vi "Pull Behavior_MWMATHIS.vi"(7 "Water Reward File":path=path "C:/Users/Mackenzie Amoroso/Desktop/REWARD_ente7102015") -> ()   [LabVIEW 2012] (continued)
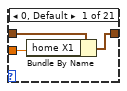
[diagram p2: hidden frame]
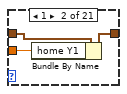
[diagram p3: hidden frame]
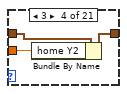
[diagram p4: hidden frame]
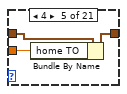
[diagram p5: hidden frame]
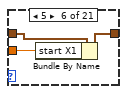
[diagram p6: hidden frame]
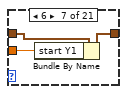
[diagram p7: hidden frame]
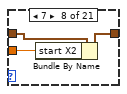
[diagram p8: hidden frame]
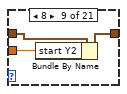
[diagram p9: hidden frame]
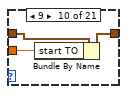
[diagram p10: hidden frame]
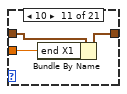
[diagram p11: hidden frame]
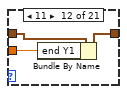
[diagram p12: hidden frame]
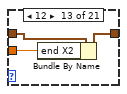
[diagram p13: hidden frame]
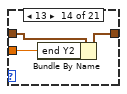
[diagram p14: hidden frame]
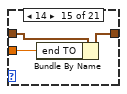
[diagram p15: hidden frame]
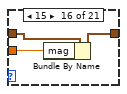
[diagram p16: hidden frame]
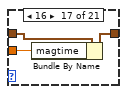
[diagram p17: hidden frame]
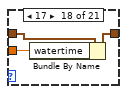
[diagram p18: hidden frame]
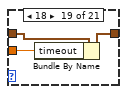
[diagram p19: hidden frame]
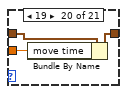
[diagram p20: hidden frame]
        n161 = Write to Binary File(file (use dialog)=w292, data=w283, 5:w279) -> (refnum out=w281:refnum<file>)  [unwired: 3 in, 2 out]
        n162 = local read "frame count 2"() -> (w278:u32)
        n163 = To Single Precision Float(number=w278) -> (single precision float=w277:sgl)
        n164 = Write to Binary File(file (use dialog)=w281, data=w277, 5:FALSE ("prepend array or string size? (T)")) -> (refnum out=w280:refnum<file>)  [unwired: 3 in, 2 out]
        n165 = local read "trial queue"() -> (w288:refnum<queue>)
        n166 = Dequeue Element(queue=w288) -> (element=w287:i32)  [unwired: 2 in, 3 out]
        n167 = To Single Precision Float(number=w287) -> (single precision float=w289:sgl)
        n168 = Write to Binary File(file (use dialog)=w280, data=w289, 5:w279) -> (refnum out=w290:refnum<file>)  [unwired: 3 in, 2 out]
        n169 = node-c288(w294) -> ()  [unwired: 1 out]
      }
      frame True {
      }
    }
    n170 = local read "stop"() -> (w275:bool)
  }
  n171 = local read "exp para array"() -> (w8:T1)
  n172 = while {
    tunnel: w30 -> [w328]
    tunnel: w27 -> [w331]
    tunnel: [w330] -> w26
    tunnel: w8 -> [w325]
    stop <- w332 stop-if-true
    # "on occurance signal give water"
    n173 = Wait on Occurrence(1:TRUE ("ignore previous (T)"), 2:w328, 3:100 ("ms timeout (-1)")) -> (0:w329:bool)
    n174 = local read "Trial #"() -> (w324:dbl)
    n175 = Index Array(array=w325, index=w324) -> (element=w323:T2)
    n176 = Unbundle By Name(w323) -> ("watertime"=w322:dbl)
    n177 = case shown="False" w329 {
      tunnel: w331 -> [w335 w361]
      tunnel: [w334 w361] -> w330
      tunnel: w322 -> [w333 _]
      frame False {
        n178 = node-c288() -> (w337:T4)  [unwired: 4 in]
        n179 = timed-sequence {
          timing: w337 -> [_]
          timing-out: [_] -> w336
          tunnel: w335 -> [w340]
          tunnel: [w339] -> w334
          tunnel: w333 -> [w338]
          n180 = timed-flat-sequence {
            tunnel: w340 -> [w348]
            tunnel: [w343] -> w339
            tunnel: w338 -> [w345]
            frame #0 {
              n181 = node-c288() -> ()  [unwired: 1 in, 1 out]
              n182 = local read "queue loop"() -> (w346:i32)
              n183 = local read "frame count 2"() -> (w341:u32)
              n184 = Write to Binary File(file (use dialog)=w348, data=w346, 5:FALSE ("prepend array or string size? (T)")) -> (refnum out=w344:refnum<file>)  [unwired: 3 in, 2 out]
              n185 = Write to Binary File(file (use dialog)=w344, data=w341, 5:FALSE ("prepend array or string size? (T)")) -> (refnum out=w343:refnum<file>)  [unwired: 3 in, 2 out]
              n186 = call-poly <vilib>:"DAQmx Write.vi"("task/channels in"=refnum<k21> "water", "data"=TRUE) -> ()  [unwired: 11 in, 3 out]
              n187 = node-c288(w345) -> ()  [unwired: 1 out]
            }
            frame #1 {
              n188 = node-c288() -> ()  [unwired: 1 in]
              n189 = node-c288() -> ()  [unwired: 1 in, 1 out]
              n190 = call-poly <vilib>:"DAQmx Write.vi"("task/channels in"=refnum<k21> "water", "data"=FALSE) -> ()  [unwired: 11 in, 3 out]
            }
          }
        }
        n191 = node-c288(w336) -> ()  [unwired: 1 out]
      }
      frame True {
      }
    }
    n192 = local read "stop"() -> (w332:bool)
  }
  n193 = Close File(refnum=w26) -> ()  [unwired: 1 in, 2 out]
  n194 = Close File(refnum=w21) -> ()  [unwired: 1 in, 2 out]
  n195 = call <vilib>:"DAQmx Stop Task.vi"("task/channels in"=w36) -> ("task out"=w39:refnum<k21>, "error out"=w38:errorcluster)  [unwired: 13 in]
  n196 = call <vilib>:"DAQmx Clear Task.vi"("task in"=w39, "error in"=w38) -> ()  [unwired: 13 in, 1 out]
  n197 = Release Queue(queue=w40) -> ()  [unwired: 2 in, 3 out]
  "Trial #" <- 0.0 ("Trial #")
  "in box begin" <- u32 4294967295 ("in box begin")
  "in trigROI" <- FALSE ("in box")
  "frame count 2" <- u32 0 ("frame count")
